vi "chart axis set position.vi"(8 "error in (no error)":errorcluster, 10 "position":u8, 11 "axis":u32) -> (0 "error out":errorcluster)   [LabVIEW 2015, in "xlsxwriter.lvlib"]
doc: "void chart_axis_set_position(lxw_chart_axis axis, uint8_t position);"
uses:
  xlsxwriter.lvlib
  xlsxwriter.dll
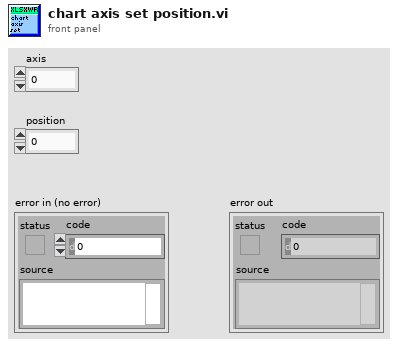
[diagram p1: front panel]
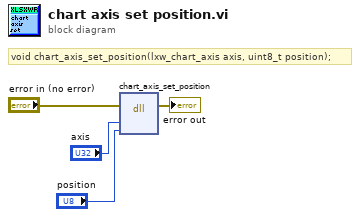
[diagram p0: block diagram]
diagram:
  # "void chart_axis_set_position(lxw_chart_axis axis, uint8_t position);"
  n1 = dll-call lib="C:/Users/WDAGUtilityAccount/Desktop/lv_vis_added_cell/xlsxwriter.*" fn="chart_axis_set_position"(error in="error in (no error)", "axis"="axis", "position"="position") -> (error out=→"error out":errorcluster)  [unwired: 5 in, 1 out]
